vi "addReshape.vi"(2 "ptr":i64, 3 "error in (no error)":errorcluster) -> (0 "ptr out":i64, 1 "error out":errorcluster)   [LabVIEW 2016, in "CNet.lvlib"]
uses:
  CNet.lvlib
  Users/jg754/Documents/Visual Studio 2015/Projects/CLearn/x64/Release/CLearn.dll
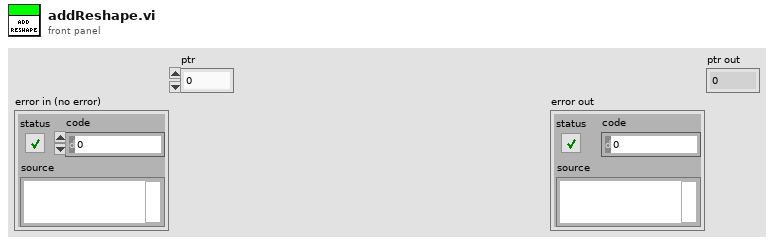
[diagram p1: front panel]
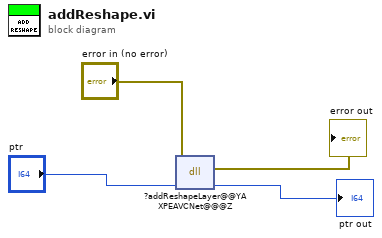
[diagram p0: block diagram]
diagram:
  n1 = dll-call lib="C:/Users/jg754/Documents/Visual Studio 2015/Projects/CLearn/x64/Release/CLearn.dll" fn="?addReshapeLayer@@YAXPEAVCNet@@@Z"(error in="error in (no error)", "ptr"="ptr") -> (error out=→"error out":errorcluster, "ptr"=→"ptr out":i64)  [unwired: 3 in, 1 out]
